vi "Main.vi"() -> ()   [LabVIEW 2023]
uses:
  <vilib>/addons/VeriStand Custom Device Scripting APIs/Data Sharing Framework/DSF Core.lvlibp/Typedefs/DSF Engine Framework Configuration.ctl
  <vilib>/addons/VeriStand Custom Device Scripting APIs/Data Sharing Framework/DSF Core.lvlibp/Typedefs/DSF Engine Plugin Configuration.ctl
  <vilib>/addons/VeriStand Custom Device Scripting APIs/Data Sharing Framework/DSF Core.lvlibp/Typedefs/Core Plugin Configuration.ctl
  <vilib>/addons/VeriStand Custom Device Scripting APIs/Data Sharing Framework/DSF Core.lvlibp/Typedefs/DSF Timing Info.ctl
  <vilib>/addons/VeriStand Custom Device Scripting APIs/Data Sharing Framework/DSF Core.lvlibp/Typedefs/DSF Settings Info.ctl
  <vilib>/addons/VeriStand Custom Device Scripting APIs/Data Sharing Framework/DSF Core.lvlibp/Typedefs/DSF Engine Plugin Thread Configuration.ctl
  <vilib>/addons/VeriStand Custom Device Scripting APIs/Data Sharing Framework/DSF Core.lvlibp/Typedefs/Core Thread Configuration.ctl
  <vilib>/addons/VeriStand Custom Device Scripting APIs/Data Sharing Framework/DSF Core.lvlibp/Typedefs/DSF Engine Transfer Group Configuration.ctl
  <vilib>/addons/VeriStand Custom Device Scripting APIs/Data Sharing Framework/DSF Core.lvlibp/Typedefs/Core Group Configuration.ctl
  <vilib>/addons/VeriStand Custom Device Scripting APIs/Data Sharing Framework/DSF Core.lvlibp/Typedefs/DSF Direction.ctl
  <vilib>/addons/VeriStand Custom Device Scripting APIs/Data Sharing Framework/DSF Core.lvlibp/Typedefs/DSF Timeout Behavior.ctl
  <vilib>/addons/VeriStand Custom Device Scripting APIs/Data Sharing Framework/DSF Core.lvlibp/Typedefs/DSF Engine Transfer Configuration.ctl
  <vilib>/addons/VeriStand Custom Device Scripting APIs/Data Sharing Framework/DSF Core.lvlibp/Typedefs/Core Transfer Configuration.ctl
  <vilib>/addons/VeriStand Custom Device Scripting APIs/Data Sharing Framework/DSF Core.lvlibp/Typedefs/DSF Engine Channel Configuration.ctl
  <vilib>/addons/VeriStand Custom Device Scripting APIs/Data Sharing Framework/DSF Core.lvlibp/Typedefs/Core Channel Configuration.ctl
  <vilib>/addons/VeriStand Custom Device Scripting APIs/Data Sharing Framework/DSF Core.lvlibp/Typedefs/DSF Data Type.ctl
  <userlib>/_OpenG.lib/array/array.llb/Index 1D Array Elements (String)__ogtk.vi
  <userlib>/_OpenG.lib/array/array.llb/Remove Duplicates from 1D Array (String)__ogtk.vi
  <userlib>/_OpenG.lib/array/array.llb/Filter 1D Array with Scalar (String)__ogtk.vi
  <vilib>/addons/VeriStand Custom Device Scripting APIs/Data Sharing Framework/DSF Core.lvlibp
  <vilib>/addons/VeriStand Custom Device Scripting APIs/Data Sharing Framework/DSF Core.lvlibp/Classes/Configuration/Core/Channel/Channel Configuration.lvclass
  <vilib>/addons/VeriStand Custom Device Scripting APIs/Data Sharing Framework/DSF Core.lvlibp/Classes/Configuration/Core/Plugin/Plugin Configuration.lvclass
  <vilib>/addons/VeriStand Custom Device Scripting APIs/Data Sharing Framework/DSF Core.lvlibp/Classes/Configuration/Core/Thread/Thread Configuration.lvclass
  <vilib>/addons/VeriStand Custom Device Scripting APIs/Data Sharing Framework/DSF Core.lvlibp/Classes/Configuration/Core/Group/Group Configuration.lvclass
  <vilib>/addons/VeriStand Custom Device Scripting APIs/Data Sharing Framework/DSF Core.lvlibp/Classes/Configuration/Core/Transfer/Transfer Configuration.lvclass
panel:
  in  "Tab Control":enum32{"Main", "Raw Data", "Raw JSON"}(tab)
  out "DSF Clusters":T1[](array[typedef])
  out "Target Sources":string[](array[string])
  out "Channel Names":string[](array[string])
  out "Channel Units":string[](array[string])
  out "Channel Types":string[](array[string])
  out "Target Destinations":string[][](array[string])
  out "JSON Strings":string[](array[string])
  out "IP Addresses":string[](array[string])
  out "Target Names":string[](array[string])
  in  "File Path Control":path
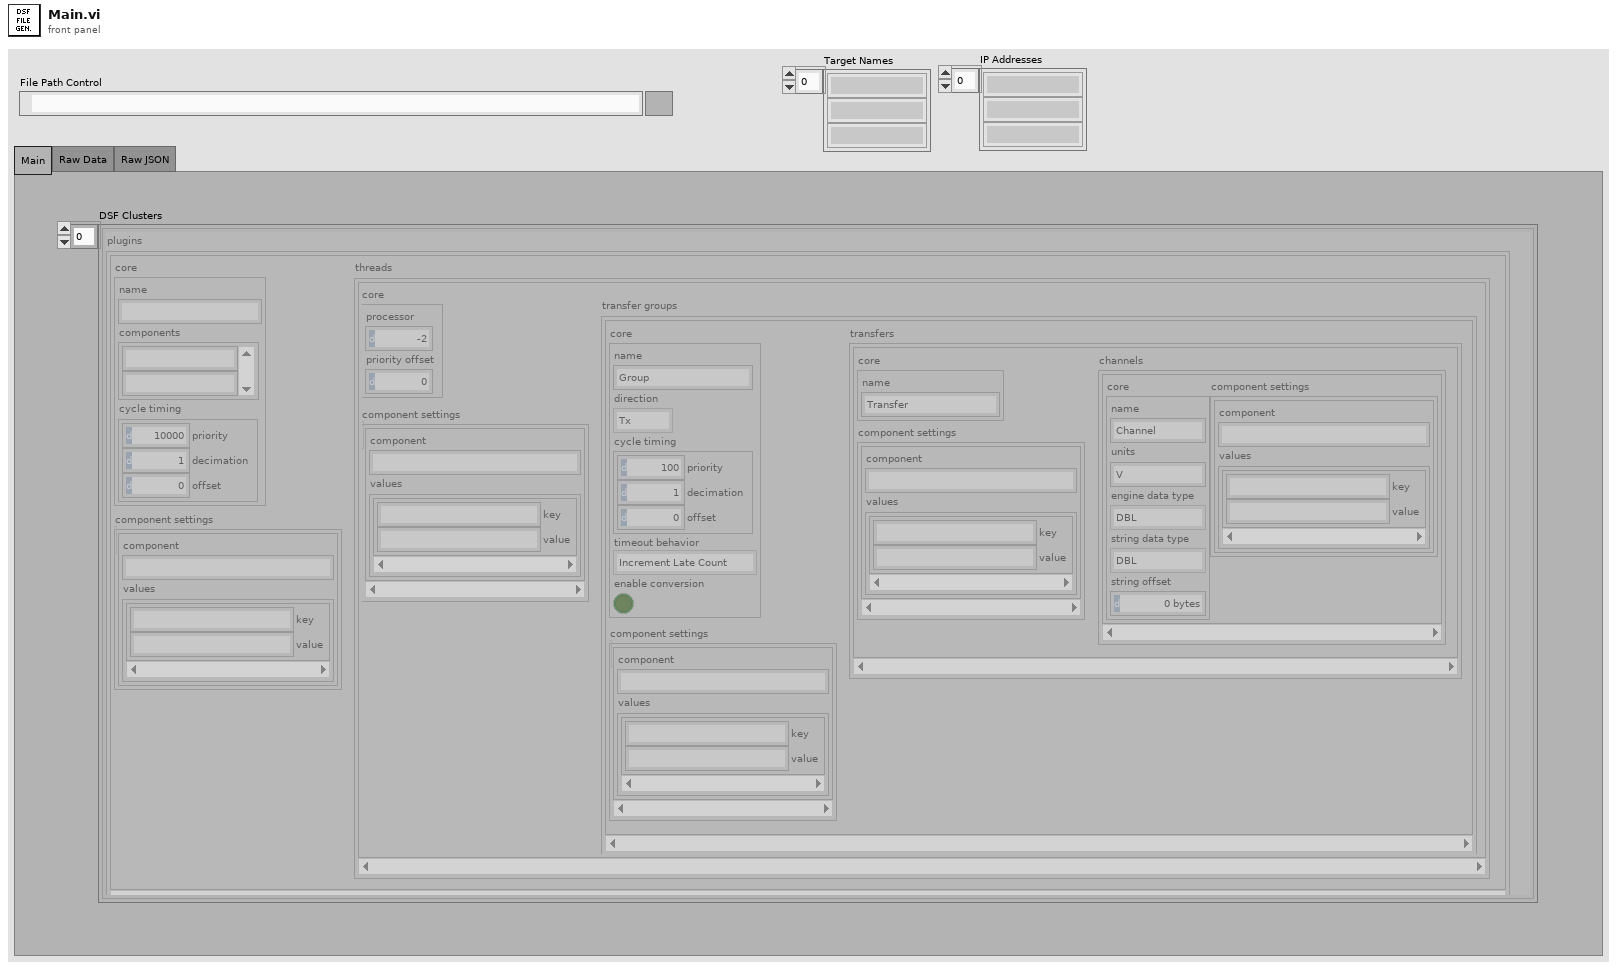
[diagram p1: front panel]
types:
  T1 = typedef "DSF Core.lvlibp/DSF Engine Framework Configuration.ctl" = cluster{"plugins":T2[]}
  T2 = typedef "DSF Core.lvlibp/DSF Engine Plugin Configuration.ctl" = cluster{"core":T3, "component settings":T5[], "threads":T6[]}
  T3 = typedef "DSF Core.lvlibp/Plugin Configuration.lvclass/Core Plugin Configuration.ctl" = cluster{"name":string, "components":string[], "cycle timing":T4}
  T4 = typedef "DSF Core.lvlibp/DSF Timing Info.ctl" = cluster{"priority":u64, "decimation":u64, "offset":u64}
  T5 = typedef "DSF Core.lvlibp/DSF Settings Info.ctl" = cluster{"component":string, "values":cluster{"key":string, "value":string}[]}
  T6 = typedef "DSF Core.lvlibp/DSF Engine Plugin Thread Configuration.ctl" = cluster{"core":T7, "component settings":T5[], "transfer groups":T8[]}
  T7 = typedef "DSF Core.lvlibp/Thread Configuration.lvclass/Core Thread Configuration.ctl" = cluster{"processor":i32, "priority offset":i16}
  T8 = typedef "DSF Core.lvlibp/DSF Engine Transfer Group Configuration.ctl" = cluster{"core":T9, "component settings":T5[], "transfers":T12[]}
  T9 = typedef "DSF Core.lvlibp/Group Configuration.lvclass/Core Group Configuration.ctl" = cluster{"name":string, "direction":T10, "cycle timing":T4, "timeout behavior":T11, "enable conversion":bool}
  T10 = typedef "DSF Core.lvlibp/DSF Direction.ctl" = enum8{"Tx", "Rx"}
  T11 = typedef "DSF Core.lvlibp/DSF Timeout Behavior.ctl" = enum8{"Increment Late Count", "Throw Error"}
  T12 = typedef "DSF Core.lvlibp/DSF Engine Transfer Configuration.ctl" = cluster{"core":T13, "component settings":T5[], "channels":T14[]}
  T13 = typedef "DSF Core.lvlibp/Transfer Configuration.lvclass/Core Transfer Configuration.ctl" = cluster{"name":string}
  T14 = typedef "DSF Core.lvlibp/DSF Engine Channel Configuration.ctl" = cluster{"core":T15, "component settings":T5[]}
  T15 = typedef "DSF Core.lvlibp/Channel Configuration.lvclass/Core Channel Configuration.ctl" = cluster{"name":string, "units":string, "engine data type":T16, "string data type":T16, "string offset":u64}
  T16 = typedef "DSF Core.lvlibp/DSF Data Type.ctl" = enum8{"Bool", "SGL", "DBL", "I8", "I16", "I32", "I64", "U8", "U16", "U32", "U64"}
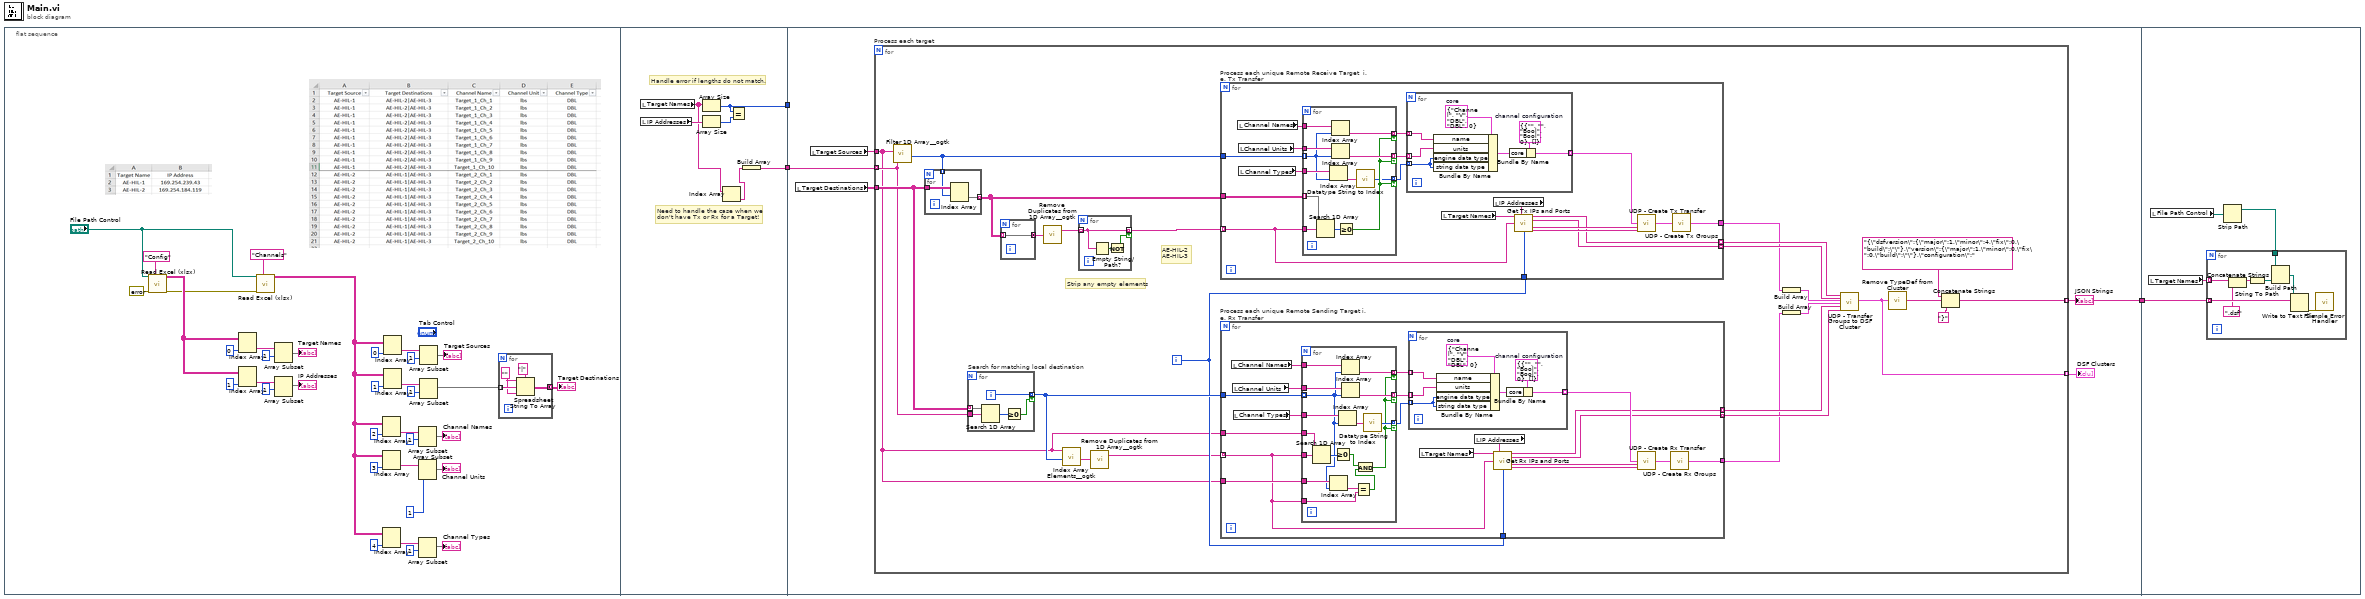
[diagram p0: block diagram]
diagram:
  n1 = flat-sequence {
    tunnel: [w48] -> w3
    tunnel: [w44] -> w2
    tunnel: w3 -> [_]
    tunnel: w2 -> [w54]
    tunnel: [w50] -> w1
    tunnel: w1 -> [w176]
    frame #0 {
      n2 = call "Read Excel (xlsx).vi"("Excel._SheetName"="Config", "error in (no error)"=errorcluster {"status"=FALSE, "code"=0, "source"=""}, "File Path Control"="File Path Control") -> ("error out"=w9:errorcluster, "data"=w10:string[][])  [unwired: 7 in]
      n3 = Index Array(array=w10, index (col)=0 ("disabled index (col)")) -> (element=w37:string[])  [unwired: 1 in]
      n4 = Index Array(array=w10, index (col)=1 ("disabled index (col)")) -> (element=w33:string[])  [unwired: 1 in]
      n5 = call "Read Excel (xlsx).vi"("Excel._SheetName"="Channels", "error in (no error)"=w9, "File Path Control"="File Path Control") -> ("data"=w8:string[][])  [unwired: 7 in, 1 out]
      n6 = Array Subset(array=w37, index=1) -> (→"Target Names":string[])  [unwired: 1 in]
      n7 = Array Subset(array=w33, index=1) -> (→"IP Addresses":string[])  [unwired: 1 in]
      n8 = Index Array(array=w8, index (col)=2 ("disabled index (col)")) -> (element=w22:string[])  [unwired: 1 in]
      n9 = Index Array(array=w8, index (col)=3 ("disabled index (col)")) -> (element=w18:string[])  [unwired: 1 in]
      n10 = Index Array(array=w8, index (col)=4 ("disabled index (col)")) -> (element=w14:string[])  [unwired: 1 in]
      n11 = Index Array(array=w8, index (col)=0 ("disabled index (col)")) -> (element=w29:string[])  [unwired: 1 in]
      n12 = Index Array(array=w8, index (col)=1 ("disabled index (col)")) -> (element=w25:string[])  [unwired: 1 in]
      n13 = Array Subset(array=w22, index=1) -> (→"Channel Names":string[])  [unwired: 1 in]
      n14 = Array Subset(array=w18, index=1) -> (→"Channel Units":string[])  [unwired: 1 in]
      n15 = Array Subset(array=w14, index=1) -> (→"Channel Types":string[])  [unwired: 1 in]
      n16 = Array Subset(array=w29, index=1) -> (→"Target Sources":string[])  [unwired: 1 in]
      n17 = Array Subset(array=w25, index=1) -> (w5:string[])  [unwired: 1 in]
      n18 = for {
        tunnel: w5 -> [w43] mode=indexing
        tunnel: [w41] -> w4 mode=concatenating
        w40 = ""
        n19 = Spreadsheet String To Array(delimiter (Tab)="|", format string=w40, spreadsheet string=w43, array type (2D Dbl)=w40) -> (array=w41:string[][])
      }
      "Target Destinations" <- w4
    }
    frame #1 {
      # "Need to handle the case when we \ndon't have Tx or Rx for a Target!"
      # "Handle error if lengths do not match."
      n20 = local read "Target Names"() -> (w46:string[])
      n21 = local read "IP Addresses"() -> (w47:string[])
      n22 = Array Size(array=w46) -> (size(s)=w48:i32)
      n23 = Array Size(array=w47) -> (size(s)=w49:i32)
      n24 = Index Array(array=w46) -> (element=w45:string)  [unwired: 1 in]
      n25 = Equal?(x=w48, y=w49) -> ()  [unwired: 1 out]
      n26 = Build Array(w45) -> (w44:string[])
    }
    frame #2 {
      n27 = local read "Target Destinations"() -> (w52:string[][])
      n28 = local read "Target Sources"() -> (w53:string[])
      n29 = for "Process each target" {
        tunnel: w54 -> [w64] mode=indexing
        tunnel: w53 -> [w63]
        tunnel: w52 -> [w73]
        tunnel: [w67] -> w50 mode=indexing
        tunnel: [w66] -> w51 mode=indexing
        i -> [w71]
        # "AE-HIL-2\nAE-HIL-3"
        # "Strip any empty elements"
        n30 = call-poly <userlib>:"Filter 1D Array__ogtk.vi"("items to filter"=w64, "array"=w63) -> ("filtered item indices"=w76:i32[])  [unwired: 4 in, 1 out]
        n31 = for {
          tunnel: w76 -> [w172] mode=indexing
          tunnel: w73 -> [w173]
          tunnel: [w171] -> w75 mode=indexing
          n32 = Index Array(array=w173, index (row)=w172) -> (element=w171:string[])  [unwired: 1 in]
        }
        n33 = for "Search for matching local destination" {
          tunnel: w73 -> [w128] mode=indexing
          tunnel: w64 -> [w127]
          tunnel: [w125] -> w72 mode=indexing if=w124
          i -> [w125]
          n34 = Search 1D Array(1D array=w128, element=w127) -> (index of element=w126:i32)  [unwired: 1 in]
          n35 = Greater Or Equal To 0?(x=w126) -> (x >= 0?=w124:bool)
        }
        n36 = for {
          tunnel: w75 -> [w170] mode=indexing
          tunnel: [w170] -> w79 mode=concatenating
        }
        n37 = call-poly <userlib>:"Remove Duplicates from 1D Array__ogtk.vi"("Input Array"=w79) -> ("Output Array"=w78:string[])  [unwired: 1 out]
        n38 = call-poly <userlib>:"Index Array Elements__ogtk.vi"("indices"=w72, "array"=w63) -> ("elements"=w74:string[])  [unwired: 9 in]
        n39 = for {
          tunnel: w78 -> [w169] mode=indexing
          tunnel: [w169] -> w77 mode=indexing if=w167
          n40 = Empty String/Path?(string/path=w169) -> (empty?=w168:bool)
          n41 = Not(x=w168) -> (.not. x?=w167:bool)
        }
        n42 = call-poly <userlib>:"Remove Duplicates from 1D Array__ogtk.vi"("Input Array"=w74) -> ("Output Array"=w65:string[])  [unwired: 1 out]
        n43 = for "Process each unique Remote Receive Target  i.e. Tx Transfer" {
          tunnel: w77 -> [w137] mode=indexing
          tunnel: w76 -> [w147]
          tunnel: w75 -> [w146]
          tunnel: w71 -> [w138]
          tunnel: [w134] -> w62 mode=indexing
          tunnel: [w133] -> w61 mode=indexing
          tunnel: [w130] -> w55
          n44 = local read "Channel Names"() -> (w145:string[])
          n45 = local read "Channel Units"() -> (w144:string[])
          n46 = local read "Channel Types"() -> (w132:string[])
          n47 = for {
            tunnel: w146 -> [w166] mode=indexing
            tunnel: w137 -> [w165]
            tunnel: w147 -> [w158] mode=indexing
            tunnel: w145 -> [w163]
            tunnel: w144 -> [w162]
            tunnel: [w161] -> w143 mode=indexing if=w157
            tunnel: [w160] -> w142 mode=indexing if=w157
            tunnel: w132 -> [w159]
            tunnel: [w155] -> w131 mode=indexing if=w157
            n48 = Search 1D Array(1D array=w166, element=w165) -> (index of element=w164:i32)  [unwired: 1 in]
            n49 = Index Array(array=w159, index=w158) -> (element=w156:string)
            n50 = Index Array(array=w163, index=w158) -> (element=w161:string)
            n51 = Index Array(array=w162, index=w158) -> (element=w160:string)
            n52 = Greater Or Equal To 0?(x=w164) -> (x >= 0?=w157:bool)
            n53 = call "Datatype String to Index.vi"("Datatype String"=w156) -> ("Datatype"=w155:T16)  [unwired: 14 in]
          }
          n54 = for {
            tunnel: w143 -> [w151] mode=indexing
            tunnel: w142 -> [w150] mode=indexing
            tunnel: [w149] -> w141 mode=indexing
            tunnel: w131 -> [w148] mode=indexing
            w152 = T15 {"name"="Channel", "units"="V", "engine data type"=enum."DBL", "string data type"=enum."DBL", "string offset"=0}  # core
            w153 = T14 {"core"={"name"="", "units"="", "engine data type"=enum."Bool", "string data type"=enum."Bool", "string offset"=0}, "component settings"=[]}  # channel configuration
            n55 = Bundle By Name(cluster=w152, "name"=w151, "units"=w150, "engine data type"=w148, "string data type"=w148) -> (w154:T15)
            n56 = Bundle By Name(cluster=w153, "core"=w154) -> (w149:T14)
          }
          n57 = local read "Target Names"() -> (w135:string[])
          n58 = local read "IP Addresses"() -> (w136:string[])
          n59 = call "Get Tx IPs and Ports.vi"("Target Names"=w135, "IP Addresses"=w136, "Remote Target Name"=w137, "Local Target Index"=w138) -> ("Local IP Address"=w134:string, "Local Port Number"=w133:string, "Remote IP Address"=w140:string, "Remote Port Number"=w139:string)  [unwired: 8 in]
          n60 = call "UDP - Create Tx Transfer.vi"("tx channels"=w141, "destination address"=w140, "destination port"=w139) -> ("Transfer"=w129:T12)  [unwired: 12 in]
          n61 = call "UDP - Create Tx Groups.vi"("Tx Transfers"=w129) -> ("Tx Transfer Group"=w130:T8)  [unwired: 14 in]
        }
        n62 = for "Process each unique Remote Sending Target i.e. Rx Transfer" {
          tunnel: w65 -> [w88] mode=indexing
          tunnel: w72 -> [w99]
          tunnel: w63 -> [w98]
          tunnel: w71 -> [w92]
          tunnel: w63 -> [w89]
          tunnel: [w87] -> w60 mode=indexing
          tunnel: [w86] -> w59 mode=indexing
          tunnel: [w81] -> w56
          n63 = local read "Channel Names"() -> (w97:string[])
          n64 = local read "Channel Units"() -> (w96:string[])
          n65 = local read "Channel Types"() -> (w82:string[])
          n66 = for {
            tunnel: w88 -> [w122]
            tunnel: w99 -> [w107] mode=indexing
            tunnel: w98 -> [w111]
            tunnel: w97 -> [w121]
            tunnel: w96 -> [w120]
            tunnel: [w119] -> w95 mode=indexing if=w109
            tunnel: [w118] -> w94 mode=indexing if=w109
            tunnel: w89 -> [w117]
            tunnel: w88 -> [w115]
            tunnel: [w110] -> w83 mode=indexing if=w109
            tunnel: w82 -> [w108]
            n67 = Search 1D Array(1D array=w111, element=w122) -> (index of element=w123:i32)  [unwired: 1 in]
            n68 = Index Array(array=w117, index=w107) -> (element=w116:string)
            n69 = Greater Or Equal To 0?(x=w123) -> (x >= 0?=w114:bool)
            n70 = Index Array(array=w108, index=w107) -> (element=w112:string)
            n71 = Index Array(array=w121, index=w107) -> (element=w119:string)
            n72 = Index Array(array=w120, index=w107) -> (element=w118:string)
            n73 = Equal?(x=w116, y=w115) -> (x = y?=w113:bool)
            n74 = And(x=w114, y=w113) -> (x .and. y?=w109:bool)
            n75 = call "Datatype String to Index.vi"("Datatype String"=w112) -> ("Datatype"=w110:T16)  [unwired: 14 in]
          }
          n76 = for {
            tunnel: w95 -> [w103] mode=indexing
            tunnel: w94 -> [w102] mode=indexing
            tunnel: [w101] -> w93 mode=indexing
            tunnel: w83 -> [w100] mode=indexing
            w104 = T15 {"name"="Channel", "units"="V", "engine data type"=enum."DBL", "string data type"=enum."DBL", "string offset"=0}  # core
            w105 = T14 {"core"={"name"="", "units"="", "engine data type"=enum."Bool", "string data type"=enum."Bool", "string offset"=0}, "component settings"=[]}  # channel configuration
            n77 = Bundle By Name(cluster=w104, "name"=w103, "units"=w102, "engine data type"=w100, "string data type"=w100) -> (w106:T15)
            n78 = Bundle By Name(cluster=w105, "core"=w106) -> (w101:T14)
          }
          n79 = local read "Target Names"() -> (w90:string[])
          n80 = local read "IP Addresses"() -> (w91:string[])
          n81 = call "Get Rx IPs and Ports.vi"("Target Names"=w90, "IP Addresses"=w91, "Remote Target Name"=w88, "Local Target Index"=w92) -> ("Local IP Address"=w87:string, "Local Port Number"=w86:string, "Remote IP Address"=w85:string, "Remote Port Number"=w84:string)  [unwired: 8 in]
          n82 = call "UDP - Create Rx Transfer.vi"("rx channels"=w93, "source address"=w85, "source port"=w84) -> ("Transfer"=w80:T12)  [unwired: 12 in]
          n83 = call "UDP - Create Rx Groups.vi"("Rx Transfers"=w80) -> ("Rx Transfer Group"=w81:T8)  [unwired: 14 in]
        }
        n84 = Build Array(w55) -> (w58:T8[])
        n85 = Build Array(w56) -> (w57:T8[])
        n86 = call "UDP - Transfer Groups to DSF Cluster.vi"("Tx local address"=w62, "Tx local port"=w61, "Tx Transfer Groups"=w58, "Rx Transfer Groups"=w57, "Rx local address"=w60, "Rx local port"=w59) -> ("DSF Cluster"=w66:T1)  [unwired: 13 in]
        n87 = call "Remove TypeDef from Cluster.vi"("configuration 1.4"=w66) -> ("JSON string"=w70:string)  [unwired: 14 in]
        n88 = Concatenate Strings("{\"dsfversion\":{\"major\":1,\"minor\":4,\"fix\":0,\"build\":\"\"},\"version\":{\"major\":1,\"minor\":0,\"fix\":0,\"build\":\"\"},\"configuration\":", w70, "}") -> (w67:string)
      }
      "JSON Strings" <- w50
      "DSF Clusters" <- w51
    }
    frame #3 {
      n89 = local read "Target Names"() -> (w175:string[])
      n90 = local read "File Path Control"() -> (w177:path)
      n91 = Strip Path(path=w177) -> (stripped path=w174:path)  [unwired: 1 out]
      n92 = for {
        tunnel: w176 -> [w185] mode=indexing
        tunnel: w175 -> [w181] mode=indexing
        tunnel: w174 -> [w184]
        n93 = Concatenate Strings(w181, ".dsf" ("string")) -> (w180:string)
        n94 = String To Path(string=w180) -> (path=w183:path)
        n95 = Build Path(base path=w184, name or relative path=w183) -> (appended path=w182:path)
        n96 = Write to Text File(file (use dialog)=w182, text=w185) -> (error out=w178:errorcluster)  [unwired: 2 in, 2 out]
        n97 = call <vilib>:"Simple Error Handler.vi"("error in (no error)"=w178) -> ()  [unwired: 4 in, 5 out]
      }
    }
  }
